vi "DSF.Engine.Memory.Buffer.Extract Channels.Preserve Value.vi"(6 "Data Type Buffers in":T6, 8 "error in (no error)":errorcluster, 9 "Channel Block":T1 {"count" format="%d elements"; "First Channel Descriptor"."VS Channel Ref" format="%016x"; "First Channel Descriptor"."Channel Parameters"."offset" format="%d bytes"}, 10 "VS Channels Array in":dbl[](array[numeric]), 11 "Buffer in":refnum<class "DSF.Engine.Memory.Buffer.lvclass">) -> (0 "error out":errorcluster, 2 "VS Channels Array out":dbl[](array[numeric]), 3 "Buffer out":refnum<class "DSF.Engine.Memory.Buffer.lvclass">, 4 "Data Type Buffers out":T6)   [LabVIEW 2016, in "DSF.Engine.lvlib" / "DSF.Engine.Memory.Buffer.lvclass"]
uses:
  DSF.Engine.Memory.Buffer.lvclass
  Typedefs/DSF.Engine.Typedefs.Type Buffers.ctl
  Shared/Typedefs/DSF.Shared.Typedefs.Configuration.Transfer.Channel Block Descriptor.ctl
  Shared/Typedefs/DSF.Shared.Typedefs.Configuration.Transfer.Channel Descriptor.ctl
  Shared/Typedefs/DSF.Shared.Typedefs.Configuration.Transfer.Channel Parameters.ctl
  Shared/Typedefs/DSF.Shared.Typedefs.Data Type.ctl
  <vilib>/NI Veristand/Custom Device API/Custom Device Item Ref.ctl
  DSF.Engine.Memory.Buffer.Read.1D.U64.vi
  DSF.Engine.Memory.Buffer.Read.1D.U32.vi
  DSF.Engine.Memory.Buffer.Read.1D.U16.vi
  DSF.Engine.Memory.Buffer.Read.1D.U8.vi
  DSF.Engine.Memory.Buffer.Read.1D.I64.vi
  DSF.Engine.Memory.Buffer.Read.1D.I32.vi
  DSF.Engine.Memory.Buffer.Read.1D.I16.vi
  DSF.Engine.Memory.Buffer.Read.1D.I8.vi
  DSF.Engine.Memory.Buffer.Read.1D.DBL.vi
  DSF.Engine.Memory.Buffer.Read.1D.SGL.vi
  DSF.Engine.Memory.Buffer.Read.1D.Bool.vi
  DSF.Shared.lvlib
  DSF.Engine.lvlib
  <vilib>/NI Veristand/Custom Device API/Custom Device API.lvlib
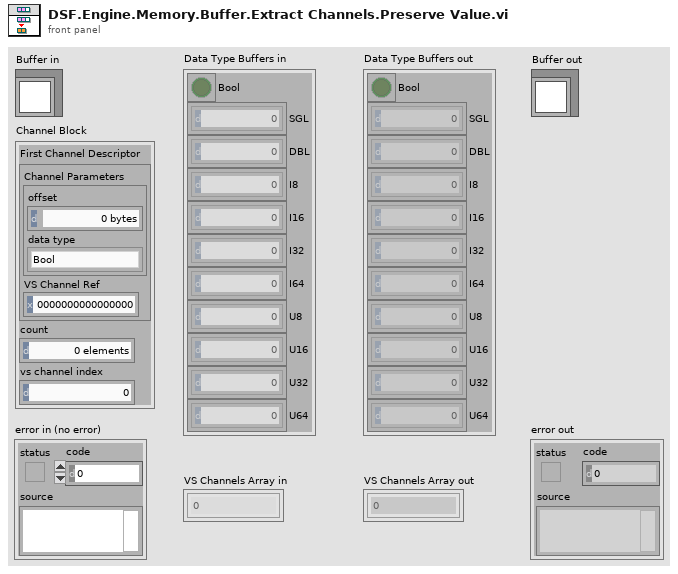
[diagram p1: front panel]
types:
  T1 = typedef "DSF.Shared.lvlib/DSF.Shared.Typedefs.Configuration.Transfer.Channel Block Descriptor.ctl" = cluster{"First Channel Descriptor":T2, "count":u64, "vs channel index":u64}
  T2 = typedef "DSF.Shared.lvlib/DSF.Shared.Typedefs.Configuration.Transfer.Channel Descriptor.ctl" = cluster{"Channel Parameters":T3, "VS Channel Ref":T5}
  T3 = typedef "DSF.Shared.lvlib/DSF.Shared.Typedefs.Configuration.Transfer.Channel Parameters.ctl" = cluster{"offset":u64, "data type":T4}
  T4 = typedef "DSF.Shared.lvlib/DSF.Shared.Typedefs.Data Type.ctl" = enum8{"Bool", "SGL", "DBL", "I8", "I16", "I32", "I64", "U8", "U16", "U32", "U64"}
  T5 = typedef "Custom Device API.lvlib/Custom Device Item Ref.ctl" = u64
  T6 = typedef "DSF.Engine.lvlib/DSF.Engine.Typedefs.Type Buffers.ctl" = cluster{"Bool":bool[], "SGL":sgl[], "DBL":dbl[], "I8":i8[], "I16":i16[], "I32":i32[], "I64":i64[], "U8":u8[], "U16":u16[], "U32":u32[], "U64":u64[]}
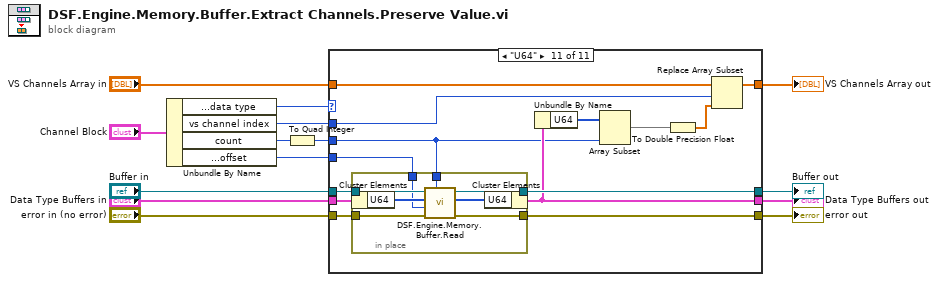
[diagram p0: block diagram]
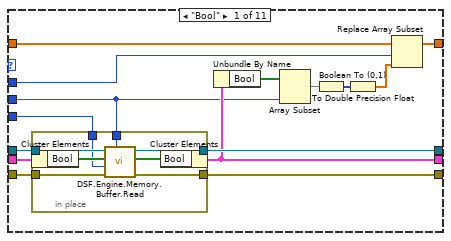
[diagram p2: hidden frame]
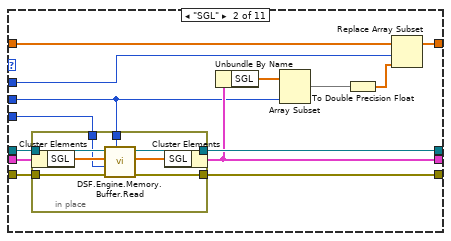
[diagram p3: hidden frame]
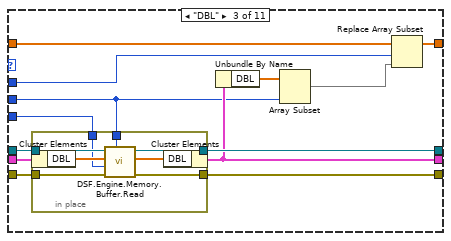
[diagram p4: hidden frame]
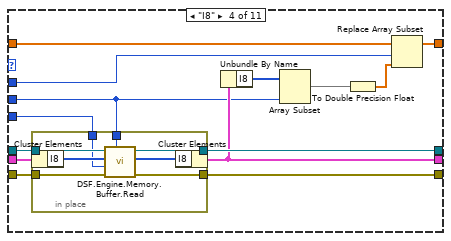
[diagram p5: hidden frame]
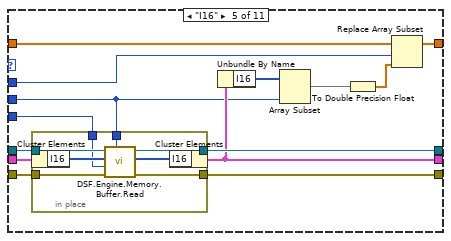
[diagram p6: hidden frame]
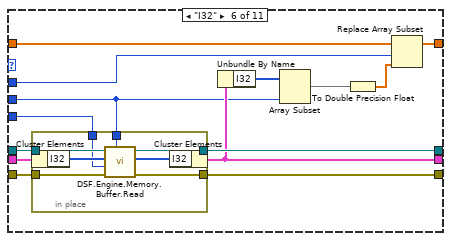
[diagram p7: hidden frame]
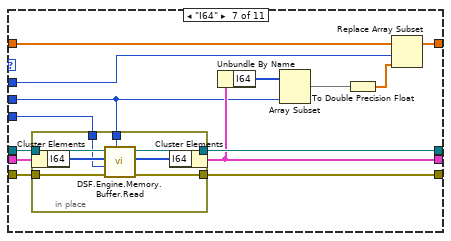
[diagram p8: hidden frame]
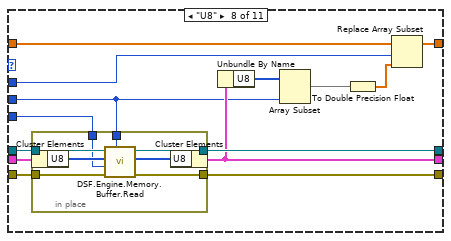
[diagram p9: hidden frame]
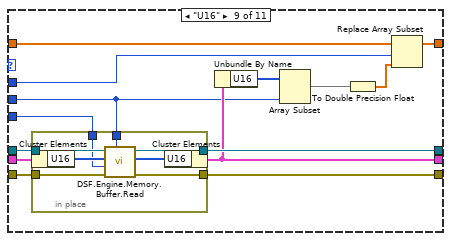
[diagram p10: hidden frame]
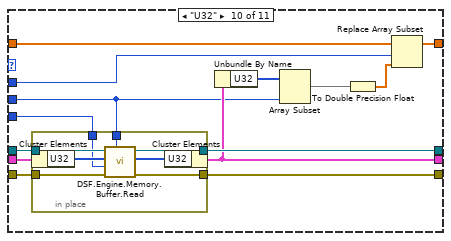
[diagram p11: hidden frame]
diagram:
  n1 = Unbundle By Name("Channel Block") -> ("First Channel Descriptor.Channel Parameters.data type"=w12:T4, "vs channel index"=w2:u64, "count"=w6:u64, "First Channel Descriptor.Channel Parameters.offset"=w7:u64)
  n2 = To Quad Integer(1:w6) -> (0:w5:i64)
  n3 = case shown="\"U64\"" w12 {
    tunnel: "Buffer in" -> [w29 w51 w72 w94 w116 w138 w160 w182 w204 w226 w248]
    tunnel: "error in (no error)" -> [w28 w50 w71 w93 w115 w137 w159 w181 w203 w225 w247]
    tunnel: [w27 w49 w70 w92 w114 w136 w158 w180 w202 w224 w246] -> w13
    tunnel: [w26 w48 w69 w91 w113 w135 w157 w179 w201 w223 w245] -> w10
    tunnel: "Data Type Buffers in" -> [w25 w47 w68 w90 w112 w134 w156 w178 w200 w222 w244]
    tunnel: [w23 w45 w66 w88 w110 w132 w154 w176 w198 w220 w242] -> w8
    tunnel: w7 -> [w24 w46 w67 w89 w111 w133 w155 w177 w199 w221 w243]
    tunnel: w5 -> [w15 w39 w61 w82 w104 w126 w148 w170 w192 w214 w236]
    tunnel: "VS Channels Array in" -> [w19 w43 w64 w86 w108 w130 w152 w174 w196 w218 w240]
    tunnel: [w18 w42 w63 w85 w107 w129 w151 w173 w195 w217 w239] -> w3
    tunnel: w2 -> [w16 w40 w62 w83 w105 w127 w149 w171 w193 w215 w237]
    frame "Bool" {
      n4 = in-place {
        in-place-border: w29 -> [w37]
        in-place-border: w28 -> [w36]
        in-place-border: [w35] -> w27
        in-place-border: w24 -> [w31]
        in-place-border: [w34] -> w26
        in-place-border: w15 -> [w30]
        n5 = in-place-cluster #1(w25) -> ("Bool"=w33:bool[])
        n6 = call-poly "DSF.Engine.Memory.Buffer.Read.vi"("count"=w30, "error in (no error)"=w36, "offset (0)"=w31, "buffer in"=w33, "Buffer in"=w37) -> ("error out"=w35:errorcluster, "buffer out"=w32:bool[], "Buffer out"=w34:refnum<class "DSF.Engine.Memory.Buffer.lvclass">)  [unwired: 3 in, 1 out]
        n7 = in-place-cluster #1("Bool"=w32) -> (w23:T6)
      }
      n8 = Unbundle By Name(w23) -> ("Bool"=w22:bool[])
      n9 = Array Subset(array=w22, length=w15) -> (w21:bool[])  [unwired: 1 in]
      n10 = Boolean To (0,1)(Boolean=w21) -> (0, 1=w20:i16[])
      n11 = To Double Precision Float(number=w20) -> (double precision float=w17:dbl[])
      n12 = Replace Array Subset(array=w19, new element=w17, index=w16) -> (w18:dbl[])
    }
    frame "SGL" {
      n13 = in-place {
        in-place-border: w51 -> [w59]
        in-place-border: w50 -> [w58]
        in-place-border: [w57] -> w49
        in-place-border: w46 -> [w53]
        in-place-border: [w56] -> w48
        in-place-border: w39 -> [w52]
        n14 = in-place-cluster #2(w47) -> ("SGL"=w55:sgl[])
        n15 = call-poly "DSF.Engine.Memory.Buffer.Read.vi"("count"=w52, "error in (no error)"=w58, "offset (0)"=w53, "buffer in"=w55, "Buffer in"=w59) -> ("error out"=w57:errorcluster, "buffer out"=w54:sgl[], "Buffer out"=w56:refnum<class "DSF.Engine.Memory.Buffer.lvclass">)  [unwired: 3 in, 1 out]
        n16 = in-place-cluster #2("SGL"=w54) -> (w45:T6)
      }
      n17 = Unbundle By Name(w45) -> ("SGL"=w44:sgl[])
      n18 = Array Subset(array=w44, length=w39) -> (w38:sgl[])  [unwired: 1 in]
      n19 = To Double Precision Float(number=w38) -> (double precision float=w41:dbl[])
      n20 = Replace Array Subset(array=w43, new element=w41, index=w40) -> (w42:dbl[])
    }
    frame "DBL" {
      n21 = in-place {
        in-place-border: w72 -> [w80]
        in-place-border: w71 -> [w79]
        in-place-border: [w78] -> w70
        in-place-border: w67 -> [w74]
        in-place-border: [w77] -> w69
        in-place-border: w61 -> [w73]
        n22 = in-place-cluster #3(w68) -> ("DBL"=w76:dbl[])
        n23 = call-poly "DSF.Engine.Memory.Buffer.Read.vi"("count"=w73, "error in (no error)"=w79, "offset (0)"=w74, "buffer in"=w76, "Buffer in"=w80) -> ("error out"=w78:errorcluster, "buffer out"=w75:dbl[], "Buffer out"=w77:refnum<class "DSF.Engine.Memory.Buffer.lvclass">)  [unwired: 3 in, 1 out]
        n24 = in-place-cluster #3("DBL"=w75) -> (w66:T6)
      }
      n25 = Unbundle By Name(w66) -> ("DBL"=w65:dbl[])
      n26 = Array Subset(array=w65, length=w61) -> (w60:dbl[])  [unwired: 1 in]
      n27 = Replace Array Subset(array=w64, new element=w60, index=w62) -> (w63:dbl[])
    }
    frame "I8" {
      n28 = in-place {
        in-place-border: w94 -> [w102]
        in-place-border: w93 -> [w101]
        in-place-border: [w100] -> w92
        in-place-border: w89 -> [w96]
        in-place-border: [w99] -> w91
        in-place-border: w82 -> [w95]
        n29 = in-place-cluster #4(w90) -> ("I8"=w98:i8[])
        n30 = call-poly "DSF.Engine.Memory.Buffer.Read.vi"("count"=w95, "error in (no error)"=w101, "offset (0)"=w96, "buffer in"=w98, "Buffer in"=w102) -> ("error out"=w100:errorcluster, "buffer out"=w97:i8[], "Buffer out"=w99:refnum<class "DSF.Engine.Memory.Buffer.lvclass">)  [unwired: 3 in, 1 out]
        n31 = in-place-cluster #4("I8"=w97) -> (w88:T6)
      }
      n32 = Unbundle By Name(w88) -> ("I8"=w87:i8[])
      n33 = Array Subset(array=w87, length=w82) -> (w81:i8[])  [unwired: 1 in]
      n34 = To Double Precision Float(number=w81) -> (double precision float=w84:dbl[])
      n35 = Replace Array Subset(array=w86, new element=w84, index=w83) -> (w85:dbl[])
    }
    frame "I16" {
      n36 = in-place {
        in-place-border: w116 -> [w124]
        in-place-border: w115 -> [w123]
        in-place-border: [w122] -> w114
        in-place-border: w111 -> [w118]
        in-place-border: [w121] -> w113
        in-place-border: w104 -> [w117]
        n37 = in-place-cluster #5(w112) -> ("I16"=w120:i16[])
        n38 = call-poly "DSF.Engine.Memory.Buffer.Read.vi"("count"=w117, "error in (no error)"=w123, "offset (0)"=w118, "buffer in"=w120, "Buffer in"=w124) -> ("error out"=w122:errorcluster, "buffer out"=w119:i16[], "Buffer out"=w121:refnum<class "DSF.Engine.Memory.Buffer.lvclass">)  [unwired: 3 in, 1 out]
        n39 = in-place-cluster #5("I16"=w119) -> (w110:T6)
      }
      n40 = Unbundle By Name(w110) -> ("I16"=w109:i16[])
      n41 = Array Subset(array=w109, length=w104) -> (w103:i16[])  [unwired: 1 in]
      n42 = To Double Precision Float(number=w103) -> (double precision float=w106:dbl[])
      n43 = Replace Array Subset(array=w108, new element=w106, index=w105) -> (w107:dbl[])
    }
    frame "I32" {
      n44 = in-place {
        in-place-border: w138 -> [w146]
        in-place-border: w137 -> [w145]
        in-place-border: [w144] -> w136
        in-place-border: w133 -> [w140]
        in-place-border: [w143] -> w135
        in-place-border: w126 -> [w139]
        n45 = in-place-cluster #6(w134) -> ("I32"=w142:i32[])
        n46 = call-poly "DSF.Engine.Memory.Buffer.Read.vi"("count"=w139, "error in (no error)"=w145, "offset (0)"=w140, "buffer in"=w142, "Buffer in"=w146) -> ("error out"=w144:errorcluster, "buffer out"=w141:i32[], "Buffer out"=w143:refnum<class "DSF.Engine.Memory.Buffer.lvclass">)  [unwired: 3 in, 1 out]
        n47 = in-place-cluster #6("I32"=w141) -> (w132:T6)
      }
      n48 = Unbundle By Name(w132) -> ("I32"=w131:i32[])
      n49 = Array Subset(array=w131, length=w126) -> (w125:i32[])  [unwired: 1 in]
      n50 = To Double Precision Float(number=w125) -> (double precision float=w128:dbl[])
      n51 = Replace Array Subset(array=w130, new element=w128, index=w127) -> (w129:dbl[])
    }
    frame "I64" {
      n52 = in-place {
        in-place-border: w160 -> [w168]
        in-place-border: w159 -> [w167]
        in-place-border: [w166] -> w158
        in-place-border: w155 -> [w162]
        in-place-border: [w165] -> w157
        in-place-border: w148 -> [w161]
        n53 = in-place-cluster #7(w156) -> ("I64"=w164:i64[])
        n54 = call-poly "DSF.Engine.Memory.Buffer.Read.vi"("count"=w161, "error in (no error)"=w167, "offset (0)"=w162, "buffer in"=w164, "Buffer in"=w168) -> ("error out"=w166:errorcluster, "buffer out"=w163:i64[], "Buffer out"=w165:refnum<class "DSF.Engine.Memory.Buffer.lvclass">)  [unwired: 3 in, 1 out]
        n55 = in-place-cluster #7("I64"=w163) -> (w154:T6)
      }
      n56 = Unbundle By Name(w154) -> ("I64"=w153:i64[])
      n57 = Array Subset(array=w153, length=w148) -> (w147:i64[])  [unwired: 1 in]
      n58 = To Double Precision Float(number=w147) -> (double precision float=w150:dbl[])
      n59 = Replace Array Subset(array=w152, new element=w150, index=w149) -> (w151:dbl[])
    }
    frame "U8" {
      n60 = in-place {
        in-place-border: w182 -> [w190]
        in-place-border: w181 -> [w189]
        in-place-border: [w188] -> w180
        in-place-border: w177 -> [w184]
        in-place-border: [w187] -> w179
        in-place-border: w170 -> [w183]
        n61 = in-place-cluster #8(w178) -> ("U8"=w186:u8[])
        n62 = call-poly "DSF.Engine.Memory.Buffer.Read.vi"("count"=w183, "error in (no error)"=w189, "offset (0)"=w184, "buffer in"=w186, "Buffer in"=w190) -> ("error out"=w188:errorcluster, "buffer out"=w185:u8[], "Buffer out"=w187:refnum<class "DSF.Engine.Memory.Buffer.lvclass">)  [unwired: 3 in, 1 out]
        n63 = in-place-cluster #8("U8"=w185) -> (w176:T6)
      }
      n64 = Unbundle By Name(w176) -> ("U8"=w175:u8[])
      n65 = Array Subset(array=w175, length=w170) -> (w169:u8[])  [unwired: 1 in]
      n66 = To Double Precision Float(number=w169) -> (double precision float=w172:dbl[])
      n67 = Replace Array Subset(array=w174, new element=w172, index=w171) -> (w173:dbl[])
    }
    frame "U16" {
      n68 = in-place {
        in-place-border: w204 -> [w212]
        in-place-border: w203 -> [w211]
        in-place-border: [w210] -> w202
        in-place-border: w199 -> [w206]
        in-place-border: [w209] -> w201
        in-place-border: w192 -> [w205]
        n69 = in-place-cluster #9(w200) -> ("U16"=w208:u16[])
        n70 = call-poly "DSF.Engine.Memory.Buffer.Read.vi"("count"=w205, "error in (no error)"=w211, "offset (0)"=w206, "buffer in"=w208, "Buffer in"=w212) -> ("error out"=w210:errorcluster, "buffer out"=w207:u16[], "Buffer out"=w209:refnum<class "DSF.Engine.Memory.Buffer.lvclass">)  [unwired: 3 in, 1 out]
        n71 = in-place-cluster #9("U16"=w207) -> (w198:T6)
      }
      n72 = Unbundle By Name(w198) -> ("U16"=w197:u16[])
      n73 = Array Subset(array=w197, length=w192) -> (w191:u16[])  [unwired: 1 in]
      n74 = To Double Precision Float(number=w191) -> (double precision float=w194:dbl[])
      n75 = Replace Array Subset(array=w196, new element=w194, index=w193) -> (w195:dbl[])
    }
    frame "U32" {
      n76 = in-place {
        in-place-border: w226 -> [w234]
        in-place-border: w225 -> [w233]
        in-place-border: [w232] -> w224
        in-place-border: w221 -> [w228]
        in-place-border: [w231] -> w223
        in-place-border: w214 -> [w227]
        n77 = in-place-cluster #10(w222) -> ("U32"=w230:u32[])
        n78 = call-poly "DSF.Engine.Memory.Buffer.Read.vi"("count"=w227, "error in (no error)"=w233, "offset (0)"=w228, "buffer in"=w230, "Buffer in"=w234) -> ("error out"=w232:errorcluster, "buffer out"=w229:u32[], "Buffer out"=w231:refnum<class "DSF.Engine.Memory.Buffer.lvclass">)  [unwired: 3 in, 1 out]
        n79 = in-place-cluster #10("U32"=w229) -> (w220:T6)
      }
      n80 = Unbundle By Name(w220) -> ("U32"=w219:u32[])
      n81 = Array Subset(array=w219, length=w214) -> (w213:u32[])  [unwired: 1 in]
      n82 = To Double Precision Float(number=w213) -> (double precision float=w216:dbl[])
      n83 = Replace Array Subset(array=w218, new element=w216, index=w215) -> (w217:dbl[])
    }
    frame "U64" {
      n84 = in-place {
        in-place-border: w248 -> [w256]
        in-place-border: w247 -> [w255]
        in-place-border: [w254] -> w246
        in-place-border: w243 -> [w250]
        in-place-border: [w253] -> w245
        in-place-border: w236 -> [w249]
        n85 = in-place-cluster #11(w244) -> ("U64"=w252:u64[])
        n86 = call-poly "DSF.Engine.Memory.Buffer.Read.vi"("count"=w249, "error in (no error)"=w255, "offset (0)"=w250, "buffer in"=w252, "Buffer in"=w256) -> ("error out"=w254:errorcluster, "buffer out"=w251:u64[], "Buffer out"=w253:refnum<class "DSF.Engine.Memory.Buffer.lvclass">)  [unwired: 3 in, 1 out]
        n87 = in-place-cluster #11("U64"=w251) -> (w242:T6)
      }
      n88 = Unbundle By Name(w242) -> ("U64"=w241:u64[])
      n89 = Array Subset(array=w241, length=w236) -> (w235:u64[])  [unwired: 1 in]
      n90 = To Double Precision Float(number=w235) -> (double precision float=w238:dbl[])
      n91 = Replace Array Subset(array=w240, new element=w238, index=w237) -> (w239:dbl[])
    }
  }
  "error out" <- w13
  "Buffer out" <- w10
  "VS Channels Array out" <- w3
  "Data Type Buffers out" <- w8
